vi "launch application batch file etc system exec.vi"(0 "Path of Program to Goose":path=path "C:/Program Files/Optellios/PS2300") -> ()   [LabVIEW 2020]
panel:
  out "concatenated string":string
  # "Browse"
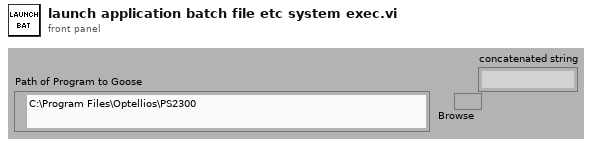
[diagram p1: front panel]
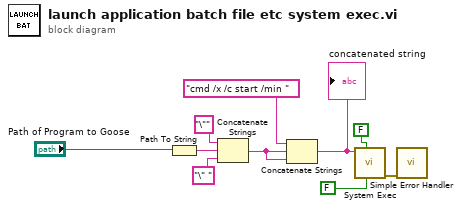
[diagram p0: block diagram]
diagram:
  n1 = Path To String(path="Path of Program to Goose") -> (string=w8:string)
  n2 = Concatenate Strings("\"" ("Substring"), w8, "\" " ("Substring")) -> (w3:string)
  n3 = Concatenate Strings("cmd /x /c start /min ", w3, w3) -> (w1:string)
  "concatenated string" <- w1
  n4 = call <vilib>:"System Exec.vi"("run minimized? (F)"=FALSE, "wait until completion? (T)"=FALSE ("Wait until done"), "command line"=w1) -> ("error out"=w5:errorcluster)  [unwired: 5 in, 3 out]
  n5 = call <vilib>:"Simple Error Handler.vi"("error in (no error)"=w5) -> ()  [unwired: 4 in, 5 out]
